vi "Receive Thread.vi"(11 "ChIndex":i32) -> ()   [LabVIEW 2018, in "CAN FD.lvlib"]
uses:
  CAN FD.lvlib
  SubVI/zlgcan.lvlib
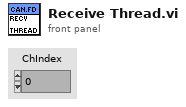
[diagram p1: front panel]
types:
  T1 = cluster{u32, u8, u8, u8, u8, cluster{"[0]":u8, "[1]":u8, "[2]":u8, "[3]":u8, "[4]":u8, "[5]":u8, "[6]":u8, "[7]":u8, "[8]":u8, "[9]":u8, "[10]":u8, "[11]":u8, "[12]":u8, "[13]":u8, "[14]":u8, "[15]":u8, "[16]":u8, "[17]":u8, "[18]":u8, "[19]":u8, "[20]":u8, "[21]":u8, "[22]":u8, "[23]":u8, "[24]":u8, "[25]":u8, "[26]":u8, "[27]":u8, "[28]":u8, "[29]":u8, "[30]":u8, "[31]":u8, "[32]":u8, "[33]":u8, "[34]":u8, "[35]":u8, "[36]":u8, "[37]":u8, "[38]":u8, "[39]":u8, "[40]":u8, "[41]":u8, "[42]":u8, "[43]":u8, "[44]":u8, "[45]":u8, "[46]":u8, "[47]":u8, "[48]":u8, "[49]":u8, "[50]":u8, "[51]":u8, "[52]":u8, "[53]":u8, "[54]":u8, "[55]":u8, "[56]":u8, "[57]":u8, "[58]":u8, "[59]":u8, "[60]":u8, "[61]":u8, "[62]":u8, "[63]":u8}, u64}[]
  T2 = cluster{u32, u8, u8, u8, u8, cluster{"[0]":u8, "[1]":u8, "[2]":u8, "[3]":u8, "[4]":u8, "[5]":u8, "[6]":u8, "[7]":u8}, u64}[]
  T3 = typedef "CAN FD.lvlib/CAN Data.ctl" = cluster{"SystemTime":timestamp, "HwTime":dbl, "Channel":u8, "ID":u32, "CANType":i16, "Direction":i16, "Remote":bool, "Ext":bool, "Len":u8, "Data":u8[], "Success":bool}
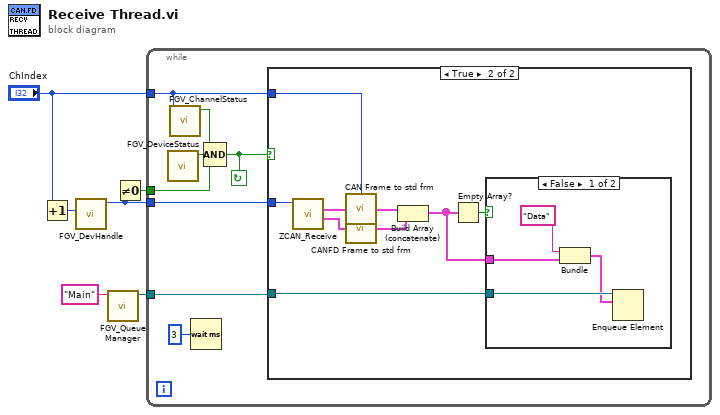
[diagram p0: block diagram]
diagram:
  n1 = Increment(x="ChIndex") -> (x+1=w3:i32)
  n2 = call "FGV_DevHandle.vi"("Type"=w3) -> ("handle out"=w2:u64)  [unwired: 8 in, 2 out]
  n3 = call "FGV_Queue Manager.vi"("Name"="Main") -> ("Queue"=w5:refnum<queue>)  [unwired: 8 in, 2 out]
  n4 = Not Equal To 0?(x=w2) -> (x != 0?=w1:bool)
  n5 = while {
    tunnel: w5 -> [w13]
    tunnel: "ChIndex" -> [w8]
    tunnel: w2 -> [w12]
    tunnel: w1 -> [w10]
    stop <- w9 continue-if-true
    n6 = call "FGV_DeviceStatus.vi"() -> ("Open?"=w11:bool)  [unwired: 10 in, 1 out]
    n7 = call "FGV_ChannelStatus.vi"("Index"=w8) -> ("Start?"=w7:bool)  [unwired: 9 in, 1 out]
    n8 = Wait (ms)(milliseconds to wait=u32 3 ("等待时间（毫秒）")) -> ()  [unwired: 1 out]
    n9 = Compound Arithmetic op=AND(w7, w11, w10) -> (w9:bool)
    n10 = case shown="True" w9 {
      tunnel: w12 -> [_ w15]
      tunnel: w8 -> [_ w21]
      tunnel: w13 -> [_ w17]
      frame False {
      }
      frame True {
        n11 = call "ZCAN_Receive.vi"("can_handle"=w15) -> ("CANFD数据帧数组"=w22:T1, "CAN数据帧数组"=w23:T2)  [unwired: 3 in, 2 out]
        n12 = call "CAN Frame to std frm.vi"("Channel"=w21, "CAN Frame"=w23) -> ("CAN Std Frm"=w20:T3[])  [unwired: 2 in]
        n13 = call "CANFD Frame to std frm.vi"("Channel"=w21, "CANFD Frame"=w22) -> ("CAN Std Frm"=w19:T3[])  [unwired: 2 in]
        n14 = Build Array (concatenate)(w20, w19) -> (w16:T3[])
        n15 = Empty Array?(array=w16) -> (empty?=w18:bool)
        n16 = case shown="False" w18 {
          tunnel: w17 -> [w27 _]
          tunnel: w16 -> [w25 _]
          frame False {
            n17 = Bundle("Data", w25) -> (w24:cluster{string, T3[]})  [unwired: 1 in]
            n18 = Enqueue Element(queue=w27, element=w24) -> ()  [unwired: 2 in, 3 out]
          }
          frame True {
          }
        }
      }
    }
  }
